vi "DecryptWaveform.vi"() -> ()   [LabVIEW 2012]
uses:
  <vilib>/Waveform/WDTFileIO.llb/ Write Waveform to File.vi
panel:
  in  "Output wav":path
  out "Output dat":path
  in  "Encrypted Message":path
  in  "Encryption":path
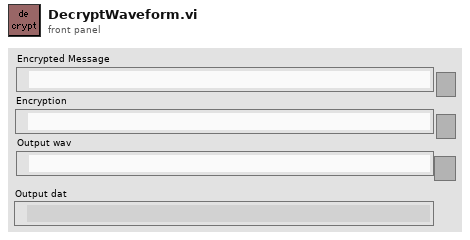
[diagram p1: front panel]
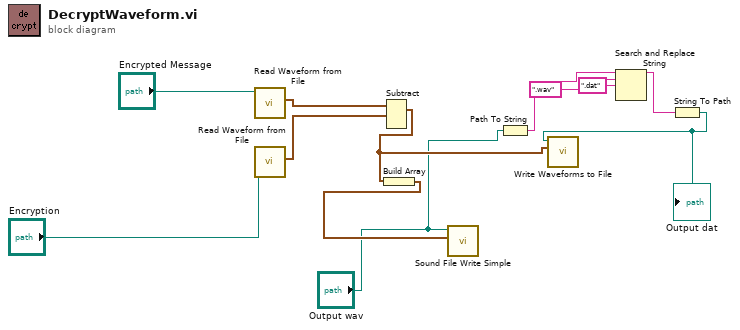
[diagram p0: block diagram]
diagram:
  n1 = call <vilib>:"Read Waveform from File.vi"("file path (dialog if empty)"="Encrypted Message") -> ("first waveform in record"=w12:waveform(dbl))  [unwired: 5 in, 3 out]
  n2 = call <vilib>:"Read Waveform from File.vi"("file path (dialog if empty)"="Encryption") -> ("first waveform in record"=w11:waveform(dbl))  [unwired: 5 in, 3 out]
  n3 = Subtract(1:w11, 2:w12) -> (0:w8:waveform(dbl))  [unwired: 1 in, 1 out]
  n4 = Build Array(w8) -> (w10:waveform(dbl)[])
  n5 = call <vilib>:"Sound File Write Simple.vi"("data"=w10, "path"="Output wav") -> ()  [unwired: 8 in, 2 out]
  n6 = Path To String(path="Output wav") -> (string=w7:string)
  n7 = Search and Replace String(input string=w7, search string=".wav" ("substring (\"\")"), replace string=".dat" ("replace string (\"\")")) -> (result string=w4:string)  [unwired: 5 in, 3 out]
  n8 = String To Path(string=w4) -> (path=w3:path)
  "Output dat" <- w3
  n9 = call-poly <vilib>:"Write Waveforms to File.vi"("waveform"=w8, "file path (dialog if empty)"=w3) -> ()  [unwired: 8 in, 2 out]
